vi "11178 UI.vi"(8 "error in (no error)":errorcluster, 11 "Node Ptr":T2 format="%.0x") -> (0 "error out":errorcluster)   [LabVIEW 2019, in "Modules.lvlib" / "11178.lvclass"]
uses:
  11178.lvclass
  <vilib>/NI VeriStand/Custom Device API/Custom Device Item Ref.ctl
  RSI Module/SubPanel Command.ctl
  C:/Users/nitest/Desktop/Git 2019/niveristand-scan-engine-module-libraries/Source/RemIO Module/RemIO Module.lvclass
  11178.lvclass/11178.ctl
  RemIO Module/RemIO Module.lvclass
  <vilib>/NI VeriStand/Custom Device API/Custom Device API.lvlib
  RSI Module/RSI Module.lvclass
panel:
  in  "Report Actuator Supply Message":enum16{"Off", "On"}(ring)
  in  "Substitute Value on Error":T1(ring)
  in  "SubPanel Event":refnum<user-event>
  in  "Header":cluster{"Section Name":string}={"Section Name"="NI REM-11178 Settings"}
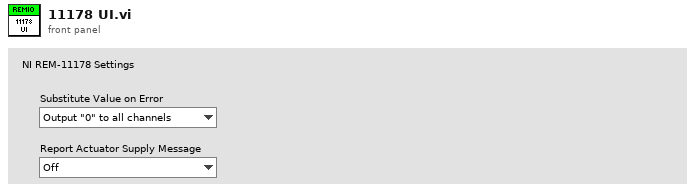
[diagram p1: front panel]
types:
  T1 = enum16{"Output \"0\" to all channels", "Hold last value"}
  T2 = typedef "Custom Device API.lvlib/Custom Device Item Ref.ctl" = u64
  T3 = typedef "NI ECAT Remote IO.lvlib/subsititute value on error.ctl" = u8
  T4 = typedef "NI ECAT Remote IO.lvlib/report supply message.ctl" = u8
  T5 = typedef "Modules.lvlib/RSI Module.lvclass/SubPanel Command.ctl" = enum16{"Stop"}
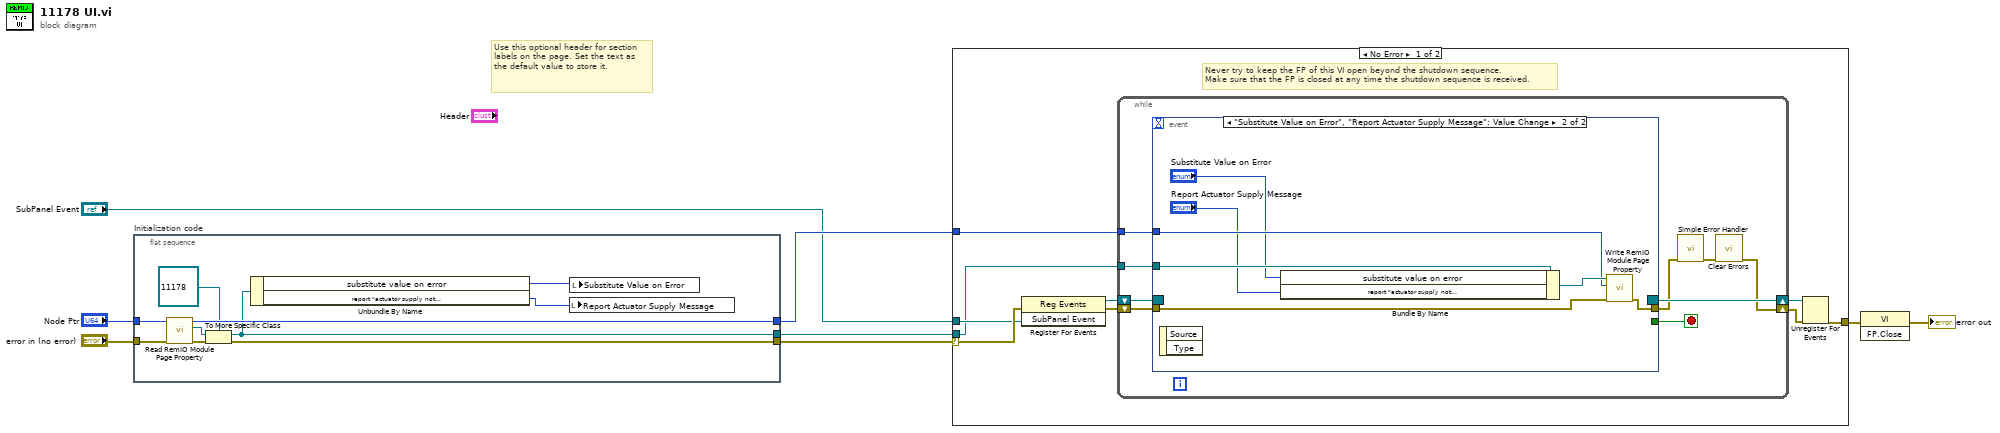
[diagram p0: block diagram]
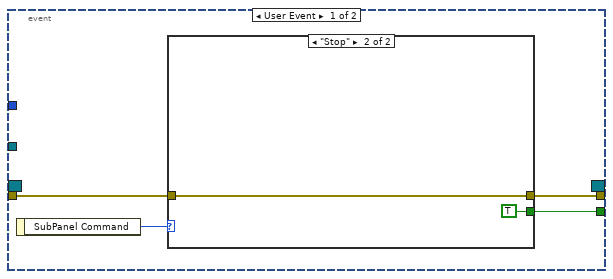
[diagram p2: hidden frame]
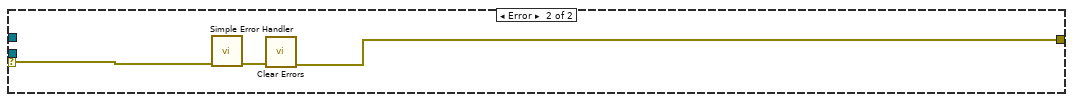
[diagram p4: hidden frame]
diagram:
  # "Use this optional header for section labels on the page. Set the text as the default value to store it."
  n1 = flat-sequence "Initialization code" {
    tunnel: "error in (no error)" -> [w17]
    tunnel: "Node Ptr" -> [w18]
    tunnel: [w13] -> w2
    tunnel: [w16] -> w5
    tunnel: [w11] -> w1
    frame #0 {
      n2 = call "Read RemIO Module Page Property.vi"("error in (no error)"=w17, "Node Ptr In"=w18) -> ("error out"=w15:errorcluster, "RemIO Module"=w14:refnum<class "RemIO Module.lvclass">, "Node Ptr Out"=w16:T2)  [unwired: 7 in]
      n3 = To More Specific Class(target class=refnum<class "11178.lvclass"> refnum ("Modules.lvlib:11178.lvclass"), reference=w14, error in=w15) -> (specific class reference=w11:refnum<class "11178.lvclass">, error out=w13:errorcluster)
      n4 = Unbundle By Name(w11) -> ("substitute value on error"=w10:T3, "report \"actuator supply not\npresent\" message?"=w9:T4)
      n5 = local write "Report Actuator Supply Message"(w9) -> ()
      n6 = local write "Substitute Value on Error"(w10) -> ()
    }
  }
  n7 = case shown="No Error" w2 {
    selector: w2 -> [w21 w53]
    tunnel: [w25 w51] -> w8
    tunnel: w5 -> [w22 _]
    tunnel: "SubPanel Event" -> [w20 _]
    tunnel: w1 -> [w19 _]
    frame No Error {
      # "Never try to keep the FP of this VI open beyond the shutdown sequence.\nMake sure that the FP is closed at any time the shutdown sequence is received."
      n8 = register-events(error in=w21, w20) -> (reference out=w23:refnum<event-registration>, error out=w24:errorcluster)  [unwired: 1 in]
      n9 = while {
        tunnel: w22 -> [w32]
        shift-right: [w29] -> w26
        shift-left: w24 -> [w35]
        shift-right: [w36] -> w27
        shift-left: w23 -> [w34]
        tunnel: w19 -> [w28]
        stop <- w33 stop-if-true
        n10 = event shown="[1] \"Substitute Value on Error\", \"Report Actuator Supply Message\": Value Change" {
          selector: w34 -> [_ _]
          dyn-events: [_ _] -> w36
          timeout: _ -> [_ _]
          tunnel: w35 -> [w39 w47]
          tunnel: [w37 _] -> w33
          tunnel: [w38 w46] -> w31
          tunnel: w32 -> [_ w48]
          tunnel: w28 -> [_ w50]
          event User Event {
            n11 = event-data() -> ("SubPanel Command"=w40:T5)  [unwired: 1 out]
            n12 = case shown="\"Stop\"" w40 {
              tunnel: w39 -> [w41 w42]
              tunnel: [w41 w42] -> w38
              tunnel: [_ TRUE] -> w37
              frame Default {
              }
              frame "Stop" {
              }
            }
          }
          event "Substitute Value on Error", "Report Actuator Supply Message": Value Change {
            n13 = event-data() -> ()  [unwired: 3 out]
            n14 = Bundle By Name(cluster=w50, "substitute value on error"="Substitute Value on Error", "report \"actuator supply not\npresent\" message?"="Report Actuator Supply Message") -> (w49:refnum<class "11178.lvclass">)
            n15 = call "Write RemIO Module Page Property.vi"("error in (no error)"=w47, "Node Ptr In"=w48, "RemIO Module"=w49) -> ("error out"=w46:errorcluster)  [unwired: 6 in, 2 out]
          }
        }
        n16 = call <vilib>:"Simple Error Handler.vi"("error in (no error)"=w31) -> ("error out"=w30:errorcluster)  [unwired: 1 in, 7 out]
        n17 = call <vilib>:"Clear Errors.vi"("error in (no error)"=w30) -> ("error out"=w29:errorcluster)  [unwired: 1 in, 5 out]
      }
      n18 = Unregister For Events(event registration refnum=w27, error in=w26) -> (error out=w25:errorcluster)
    }
    frame Error {
      n19 = call <vilib>:"Simple Error Handler.vi"("error in (no error)"=w53) -> ("error out"=w52:errorcluster)  [unwired: 1 in, 7 out]
      n20 = call <vilib>:"Clear Errors.vi"("error in (no error)"=w52) -> ("error out"=w51:errorcluster)  [unwired: 1 in, 5 out]
    }
  }
  n21 = invoke class="VI" method="FP.Close"(error in=w8) -> (error out=→"error out":errorcluster)  [unwired: 2 in, 2 out]
